vi "Read Single Measurement (Current).vi"(0 "VISA resource name":refnum<visa-resource-name>, 5 "Maximum Time (10000 ms)":i32=10000, 11 "error in (no error)":errorcluster) -> (3 "Peak Current":dbl, 4 "VISA resource name out":refnum<visa-resource-name>, 6 "DC Current":dbl, 8 "AC RMS Current":dbl, 10 "AC + DC RMS Current":dbl, 15 "error out":errorcluster)   [LabVIEW 2020, in "Agilent 681x Series.lvlib"]
doc: "Initiates and reads an instantaneous current measurement.\n\n<B>Note:</B>\n\nThis VI changes the <B>Trigger Source</B> to <B>Bus</B> and uses a software trigger after the instrument is initiated. If you want to control the triggering and other features, please use the low level VIs."
uses:
  <instrlib>/Agilent 681x Series/Agilent 681x Series.lvlib
  <instrlib>/Agilent 681x Series/Public/Data/Low Level/Fetch Single Measurement (Current).vi
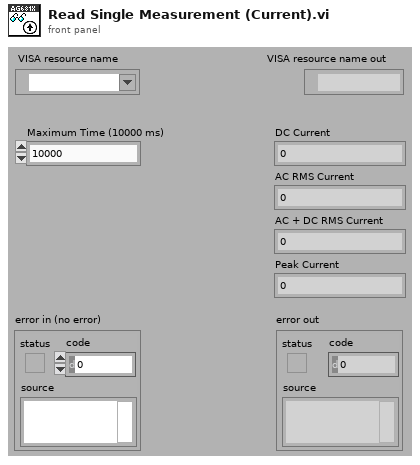
[diagram p1: front panel]
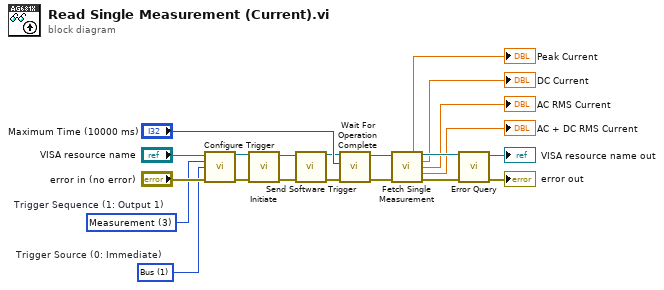
[diagram p0: block diagram]
diagram:
  w11 = 1 items=["Immediate", "Bus", "External", "Phase", "Trigger Out"]  # Trigger Source (0: Immediate)
  w12 = 3 items=["Output"=1, "Synchronous Source"=2, "Measurement"=3]  # Trigger Sequence (1: Output 1)
  n1 = call <instrlib>:"Configure Trigger.vi"("VISA resource name"="VISA resource name", "Trigger Sequence (1: Output 1)"=w12, "Trigger Source (0: Immediate)"=w11, "error in (no error)"="error in (no error)") -> ("VISA resource name out"=w9:refnum<visa-resource-name>, "error out"=w10:errorcluster)  [unwired: 10 in]
  n2 = call <instrlib>:"Initiate.vi"("error in (no error)"=w10, "VISA resource name"=w9) -> ("error out"=w8:errorcluster, "VISA resource name out"=w7:refnum<visa-resource-name>)  [unwired: 8 in]
  n3 = call <instrlib>:"Send Software Trigger.vi"("VISA resource name"=w7, "error in (no error)"=w8) -> ("VISA resource name out"=w6:refnum<visa-resource-name>, "error out"=w5:errorcluster)  [unwired: 12 in]
  n4 = call <instrlib>:"Wait For Operation Complete.vi"("error in (no error)"=w5, "Maximum Time (10000 ms)"="Maximum Time (10000 ms)", "VISA resource name"=w6) -> ("error out"=w20:errorcluster, "VISA resource name out"=w17:refnum<visa-resource-name>)  [unwired: 7 in]
  n5 = call-poly <instrlib>:"Fetch Single Measurement.vi"("VISA resource name"=w17, "error in (no error)"=w20) -> ("Peak Current"=→"Peak Current":dbl, "VISA resource name out"=w19:refnum<visa-resource-name>, "DC Current"=→"DC Current":dbl, "AC RMS Current"=→"AC RMS Current":dbl, "AC + DC RMS Current"=→"AC + DC RMS Current":dbl, "error out"=w18:errorcluster)  [unwired: 8 in]
  n6 = call <instrlib>:"Error Query.vi"("error in (no error)"=w18, "VISA resource name"=w19) -> ("error out"=→"error out":errorcluster, "VISA resource name out"=→"VISA resource name out":refnum<visa-resource-name>)  [unwired: 6 in, 2 out]
